vi "Get Table Data.vi"(8 "error in":errorcluster, 11 "Cluster in":T1={"Running VI"=refnum, "Test VI"=refnum, "Q Ref"=refnum, "UE"=refnum, "Data"=variant, "Timeout"=-1, "ListBox[]"=[], "Source Path"=path "", "Delta Time"=0.0, "ExifInfo[]"=[], "ListIndex"=0, "counter"=0, "Format"=enum."Files Only", "total"=0, "Operation"=enum."Read Info", "Status"=""} {"ExifInfo[]"."New DateTime" format="%<%.3X>T"; "ExifInfo[]"."DateTimeOrginal" format="%<%.3X>T"}) -> (0 "error out":errorcluster, 3 "Cluster out":T1={"Running VI"=refnum, "Test VI"=refnum, "Q Ref"=refnum, "UE"=refnum, "Data"=variant, "Timeout"=-1, "ListBox[]"=[], "Source Path"=path "", "Delta Time"=0.0, "ExifInfo[]"=[], "ListIndex"=0, "counter"=0, "Format"=enum."Files Only", "total"=0, "Operation"=enum."Read Info", "Status"=""} {"ExifInfo[]"."New DateTime" format="%<%.3X>T"; "ExifInfo[]"."DateTimeOrginal" format="%<%.3X>T"}, 4 "Table[]":string[][](array[string]))   [LabVIEW 2023, in "EXIF Modifier.lvlib"]
uses:
  Controls/exif_consumer cluster.ctl
  Controls/exif_info cluster.ctl
  EXIF Modifier.lvlib
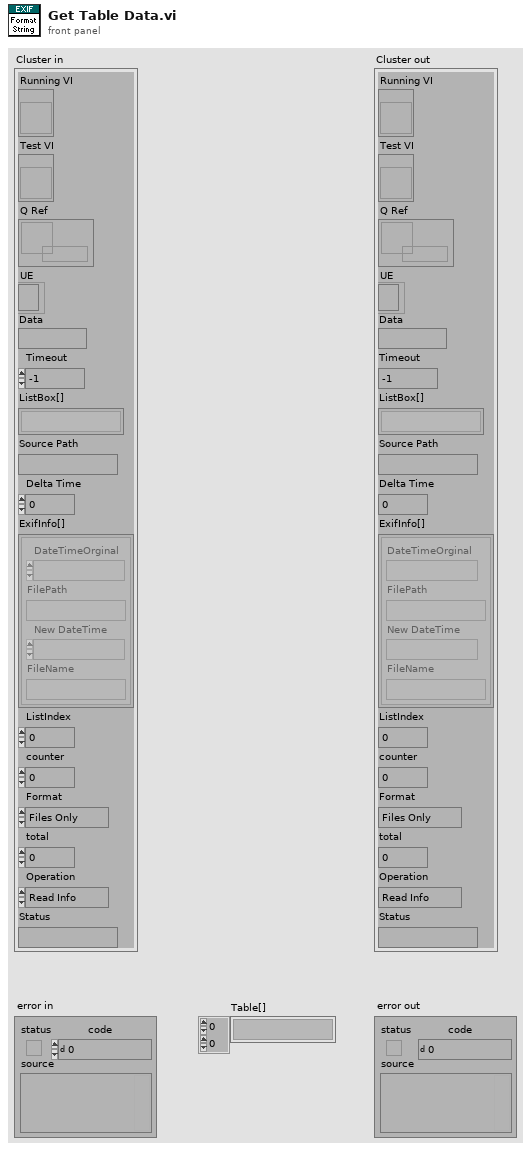
[diagram p1: front panel]
types:
  T1 = typedef "EXIF Modifier.lvlib/exif_consumer cluster.ctl" = cluster{"Running VI":refnum<vi>, "Test VI":refnum<vi>, "Q Ref":refnum<queue>, "UE":refnum<event-registration>, "Data":variant, "Timeout":i32, "ListBox[]":string[][], "Source Path":path, "Delta Time":dbl, "ExifInfo[]":T2[], "ListIndex":i32, "counter":i32, "Format":enum16{"Files Only", "Files Date", "All"}, "total":i32, "Operation":enum16{"Read Info", "Write Info"}, "Status":string}
  T2 = typedef "EXIF Modifier.lvlib/exif_info cluster.ctl" = cluster{"DateTimeOrginal":timestamp, "FilePath":path, "New DateTime":timestamp, "FileName":string}
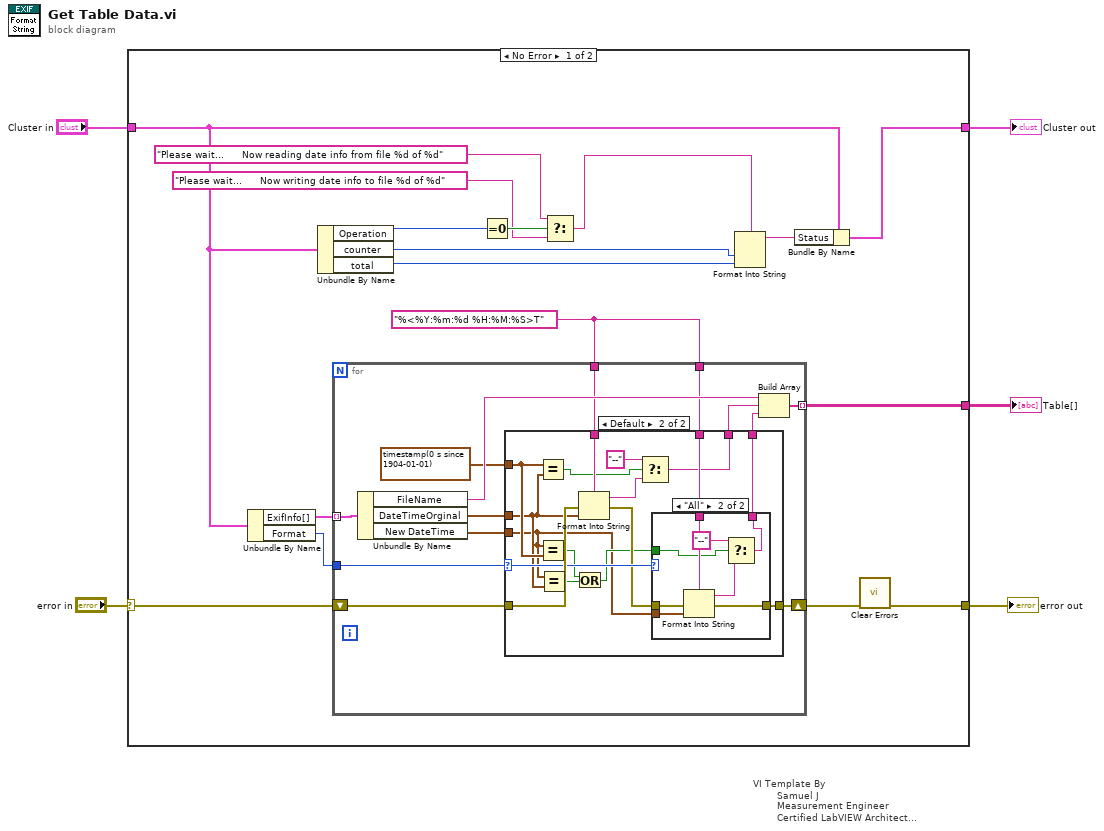
[diagram p0: block diagram]
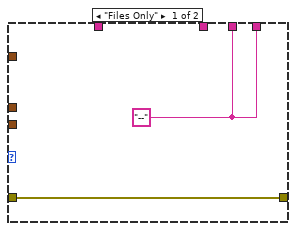
[diagram p2: hidden frame]
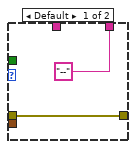
[diagram p3: hidden frame]
diagram:
  n1 = case "VI Template By\n        Samuel J\n        Measurement Engineer\n        Certified LabVIEW Architect\n        Vestas Technology R&D Chennai" shown="No Error" "error in" {
    selector: "error in" -> [w21 w66]
    tunnel: [w16 w66] -> w4
    tunnel: [w12 w65] -> w2
    tunnel: "Cluster in" -> [w13 w65]
    tunnel: [w18 _] -> w1
    frame No Error {
      w19 = "%<%Y:%m:%d %H:%M:%S>T" ("format string")
      n2 = Unbundle By Name(w13) -> ("ExifInfo[]"=w22:T2[], "Format"=w17:enum16{"Files Only", "Files Date", "All"})
      n3 = Unbundle By Name(w13) -> ("Operation"=w10:enum16{"Read Info", "Write Info"}, "counter"=w15:i32, "total"=w14:i32)
      n4 = for {
        tunnel: w22 -> [w35] mode=indexing
        shift-right: [w28] -> w20
        shift-left: w21 -> [w29]
        tunnel: w19 -> [w31]
        tunnel: w19 -> [w30]
        tunnel: [w25] -> w18 mode=indexing
        tunnel: w17 -> [w24]
        n5 = Unbundle By Name(w35) -> ("FileName"=w34:string, "DateTimeOrginal"=w33:timestamp, "New DateTime"=w32:timestamp)
        n6 = case shown="Default" w24 {
          selector: w24 -> [_ w49]
          tunnel: w33 -> [_ w42]
          tunnel: w32 -> [_ w38]
          tunnel: w31 -> [_ w54]
          tunnel: w30 -> [_ w53]
          tunnel: w29 -> [w37 w52]
          tunnel: [w37 w51] -> w28
          tunnel: [w36 w47] -> w27
          tunnel: [w36 w50] -> w26
          tunnel: timestamp(0 s since 1904-01-01) ("DateTimeOrginal") -> [_ w43]
          frame "Files Only" {
            w36 = "--"
          }
          frame Default {
            n7 = Equal?(x=w43, y=w42) -> (x = y?=w45:bool)
            n8 = Equal?(x=w38, y=w43) -> (x = y?=w40:bool)
            n9 = Equal?(x=w38, y=w42) -> (x = y?=w41:bool)
            n10 = Or(x=w40, y=w41) -> (x .or. y?=w39:bool)
            n11 = Format Into String(format string=w54, error in=w52, w42) -> (resulting string=w44:string, error out=w48:errorcluster)  [unwired: 1 in]
            n12 = Select(t="--", s=w45, f=w44) -> (s? t:f=w47:string)
            n13 = case shown="\"All\"" w49 {
              tunnel: w38 -> [_ w64]
              tunnel: w53 -> [_ w63]
              tunnel: w48 -> [w56 w62]
              tunnel: [w56 w60] -> w51
              tunnel: ["--" w58] -> w50
              tunnel: w39 -> [_ w57]
              frame Default {
              }
              frame "All" {
                n14 = Format Into String(format string=w63, error in=w62, w64) -> (resulting string=w59:string, error out=w60:errorcluster)  [unwired: 1 in]
                n15 = Select(t="--", s=w57, f=w59) -> (s? t:f=w58:string)
              }
            }
          }
        }
        n16 = Build Array(w34, w27, w26) -> (w25:string[])
      }
      n17 = Equal To 0?(x=w10) -> (x = 0?=w9:bool)
      n18 = Select(t="Please wait...      Now reading date info from file %d of %d" ("format string"), s=w9, f="Please wait...      Now writing date info to file %d of %d" ("format string")) -> (s? t:f=w6:string)
      n19 = Format Into String(format string=w6, w15, w14) -> (resulting string=w11:string)  [unwired: 2 in, 1 out]
      n20 = Bundle By Name(cluster=w13, "Status"=w11) -> (w12:T1)
      n21 = call <vilib>:"Clear Errors.vi"("error in (no error)"=w20) -> ("error out"=w16:errorcluster)  [unwired: 5 in, 1 out]
    }
    frame Error {
    }
  }
  "error out" <- w4
  "Cluster out" <- w2
  "Table[]" <- w1
